vi "DVRCreator.vi"(0 "Increment":bool, 5 "Stop":bool, 11 "Error in":errorcluster) -> (15 "Error out":errorcluster)   [LabVIEW 2020]
panel:
  # "DVR SCOPE"
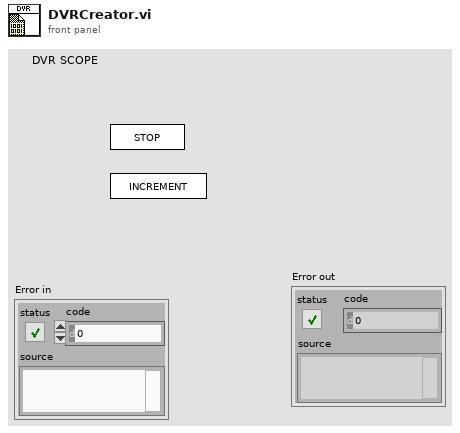
[diagram p1: front panel]
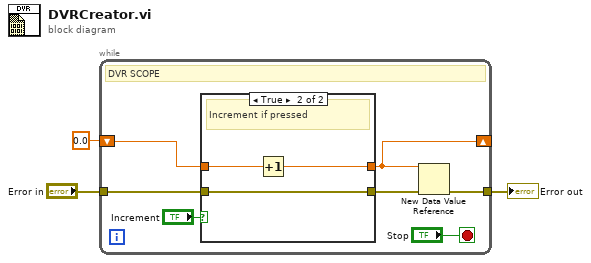
[diagram p0: block diagram]
diagram:
  n1 = while {
    tunnel: "Error in" -> [w7]
    tunnel: [w9] -> w2
    shift-right: [w4] -> _
    shift-left: 0.0 -> [w5]
    stop <- "Stop" stop-if-true
    # "DVR SCOPE"
    n2 = case shown="True" "Increment" {
      tunnel: w7 -> [w11 w15]
      tunnel: [w11 w15] -> w6
      tunnel: w5 -> [w12 w14]
      tunnel: [w12 w13] -> w4
      frame False {
        # "Continue"
      }
      frame True {
        # "Increment if pressed"
        n3 = Increment(x=w14) -> (x+1=w13:dbl)
      }
    }
    n4 = New Data Value Reference(data value=w4, error in=w6) -> (error out=w9:errorcluster)  [unwired: 1 out]
  }
  "Error out" <- w2
